vi "Quantitycheck.vi"(8 "NUM INPUT":dbl, 11 "key":string) -> ()   [LabVIEW 2018]
uses:
  <vilib>/Utility/config.llb/Read Key (Double).vi
  <vilib>/Utility/config.llb/Write Key (Double).vi
  <vilib>/Utility/config.llb/NI_LVConfig.lvlib
panel:
  out "value":u32
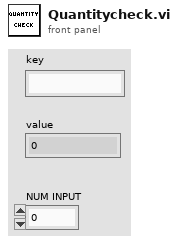
[diagram p1: front panel]
types:
  T1 = typedef "NI_LVConfig.lvlib/Config Data RefNum.ctl" = refnum<k1>
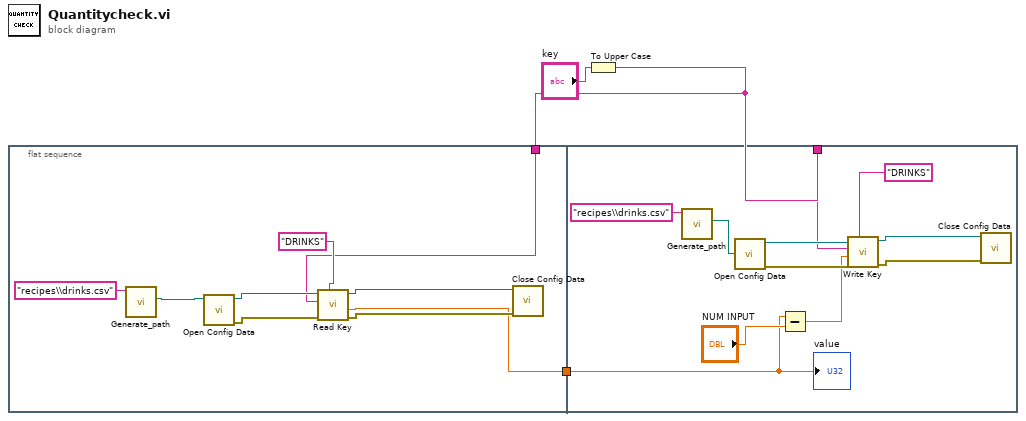
[diagram p0: block diagram]
diagram:
  n1 = flat-sequence {
    tunnel: w2 -> [w7]
    tunnel: [w6] -> w1
    tunnel: w2 -> [w18]
    tunnel: w1 -> [w15]
    frame #0 {
      n2 = call "Generate_path.vi"("name or relative path"="recipes\\drinks.csv") -> ("MyFile"=w4:path)  [unwired: 10 in]
      n3 = call <vilib>:"Open Config Data.vi"("configuration file path"=w4) -> ("error out"=w11:errorcluster, "refnum"=w9:T1)  [unwired: 8 in, 1 out]
      n4 = call-poly <vilib>:"Read Key.vi"("section"="DRINKS", "error in (no error)"=w11, "key"=w7, "refnum"=w9) -> ("error out"=w12:errorcluster, "value"=w6:dbl, "refnum out"=w10:T1)  [unwired: 4 in, 1 out]
      n5 = call <vilib>:"Close Config Data.vi"("error in (no error)"=w12, "refnum"=w10) -> ()  [unwired: 8 in, 2 out]
    }
    frame #1 {
      n6 = call "Generate_path.vi"("name or relative path"="recipes\\drinks.csv") -> ("MyFile"=w13:path)  [unwired: 10 in]
      n7 = call <vilib>:"Open Config Data.vi"("configuration file path"=w13) -> ("error out"=w22:errorcluster, "refnum"=w20:T1)  [unwired: 8 in, 1 out]
      n8 = Subtract(x=w15, y="NUM INPUT") -> (x-y=w17:dbl)
      n9 = call-poly <vilib>:"Write Key.vi"("section"="DRINKS", "error in (no error)"=w22, "value"=w17, "key"=w18, "refnum"=w20) -> ("error out"=w23:errorcluster, "refnum out"=w21:T1)  [unwired: 4 in, 1 out]
      n10 = call <vilib>:"Close Config Data.vi"("error in (no error)"=w23, "refnum"=w21) -> ()  [unwired: 8 in, 2 out]
      "value" <- w15
    }
  }
  n11 = To Upper Case(1:"key") -> (0:w2:string)
